vi "update config.vi"(8 "error in (no error)":errorcluster, 10 "user configurations":T1={"vst_device"=["VST_1", "VST_2"], "RF gain "=10.0, "buffer size"=524288, "center frequency (Hz) "=1000000000.0, "P2P sample rate"=200000000.0, "mode"=enum."5785 - 2*180MHz", "devicess"=["IF_transiver_0", "IF_transiver_1", "IF_transiver_2"], "gen for df"=FALSE, "Rx settings"={"min PW         "=0.0, "max gap        "=0.0, "detection bar"=0.0, "peak detect                        "=FALSE}}, 11 "5785_3.2GHz_one channel in":refnum<class "5785_3.2GHz_one channel.lvclass">) -> (0 "error out":errorcluster, 1 "min frequency":dbl, 2 "max frequency":dbl, 3 "5785_3.2GHz_one channel out":refnum<class "5785_3.2GHz_one channel.lvclass">)   [LabVIEW 2021, in "5785_3.2GHz_one channel.lvclass"]
uses:
  5785_3.2GHz_one channel.lvclass
  pulse_tx_vis/CTL/user config.ctl
  <vilib>/userdefined/High Color/nirio_resource_hc.ctl
  5785_3.2GHz_one channel.lvclass/5785_3.2GHz_one channel.ctl
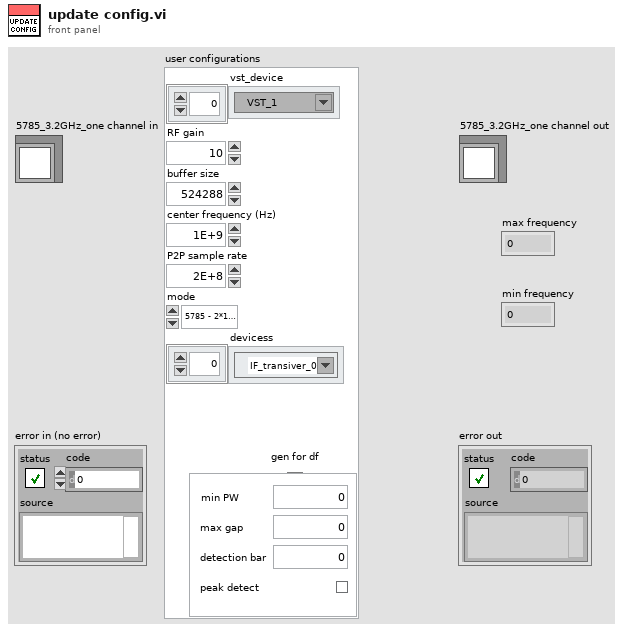
[diagram p1: front panel]
types:
  T1 = typedef "user config.ctl" = cluster{"vst_device":refnum<k15>[], "RF gain ":dbl, "buffer size":u32, "center frequency (Hz) ":dbl, "P2P sample rate":dbl, "mode":enum16{"USRP - 180MHz", "5785 - 2*180MHz", "5785 - 3.2GHz", "P2P - VST"}, "devicess":T2[], "gen for df":bool, "Rx settings":cluster{"min PW         ":dbl, "max gap        ":dbl, "detection bar":dbl, "peak detect                        ":bool}}
  T2 = typedef "nirio_resource_hc.ctl" = tag
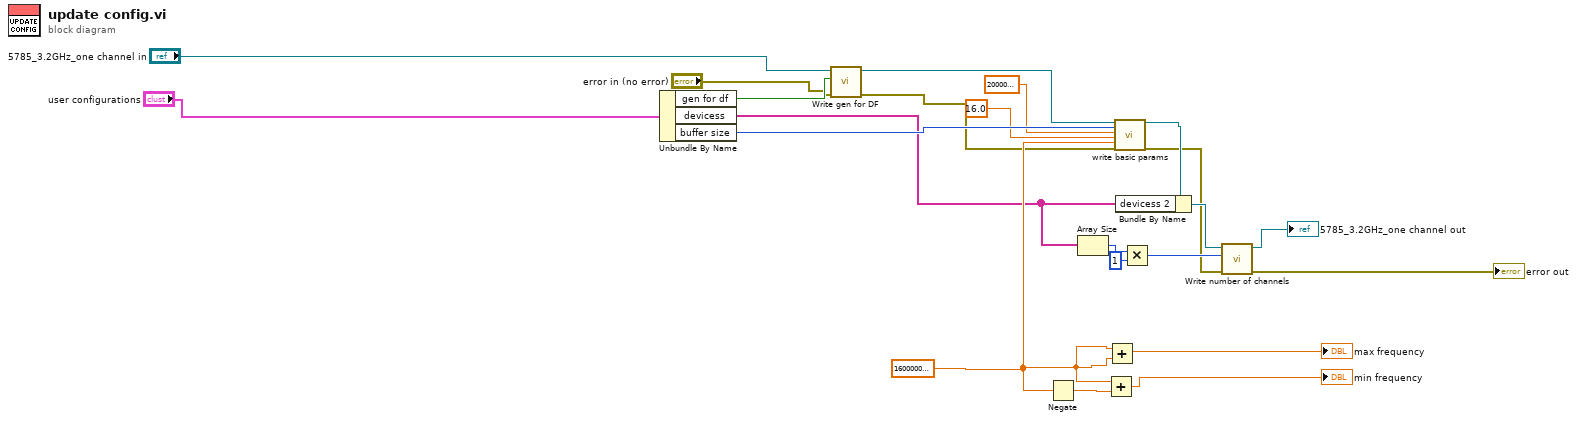
[diagram p0: block diagram]
diagram:
  w14 = 1600000000.0
  n1 = Unbundle By Name("user configurations") -> ("gen for df"=w10:bool, "devicess"=w4:T2[], "buffer size"=w17:u32)
  n2 = call-dynamic "Write gen for DF.vi"("error in (no error)"="error in (no error)", "gen for DF"=w10, "device_type in"="5785_3.2GHz_one channel in") -> ("error out"=w9:errorcluster, "device_type out"=w12:refnum<class "5785_3.2GHz_one channel.lvclass">)  [unwired: 7 in]
  n3 = Negate(x=w14) -> (-x=w21:dbl)
  n4 = Array Size(array=w4) -> (size(s)=w7:i32)
  n5 = Add(x=w14, y=w21) -> (x+y=→"min frequency":dbl)
  n6 = Add(x=w14, y=w14) -> (x+y=→"max frequency":dbl)
  n7 = call-dynamic "write basic params.vi"("device_type in"=w12, "buffer size"=w17, "Fs  FPGA"=200000000.0, "SPC"=16.0 ("Fs  FPGA"), "center frequency (Hz)"=w14, "error in (no error)"=w9) -> ("device_type out"=w13:refnum<class "5785_3.2GHz_one channel.lvclass">, "error out"=w1:errorcluster)  [unwired: 12 in]
  "error out" <- w1
  n8 = Bundle By Name(cluster=w13, "devicess 2"=w4) -> (w3:refnum<class "5785_3.2GHz_one channel.lvclass">)
  n9 = Multiply(x=w7, y=1) -> (x*y=w5:i32)
  n10 = call-dynamic "Write number of channels.vi"("error in (no error)"=w1, "number of channels"=w5, "device_type in"=w3) -> ("device_type out"=→"5785_3.2GHz_one channel out":refnum<class "5785_3.2GHz_one channel.lvclass">)  [unwired: 7 in, 1 out]
